vi "Close.vi"(8 "error in (no error)":errorcluster, 11 "SpinCoater in":refnum<class "SpinCoater.lvclass">) -> (0 "error out":errorcluster, 3 "SpinCoater out":refnum<class "SpinCoater.lvclass">)   [LabVIEW 2020, in "SpinCoater.lvclass"]
uses:
  <instrlib>/Classes/SpinCoater/SpinCoater.lvclass
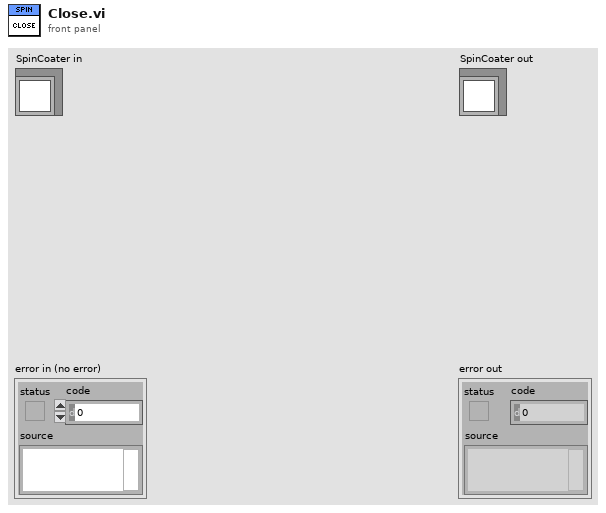
[diagram p1: front panel]
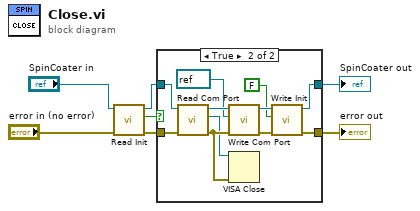
[diagram p0: block diagram]
diagram:
  n1 = call-dynamic "Read Init.vi"("error in (no error)"="error in (no error)", "SpinCoater in"="SpinCoater in") -> ("error out"=w4:errorcluster, "Init"=w3:bool, "SpinCoater out"=w5:refnum<class "SpinCoater.lvclass">)  [unwired: 7 in]
  n2 = case shown="True" w3 {
    tunnel: w5 -> [w9 w20]
    tunnel: w4 -> [w8 w19]
    tunnel: [w9 w11] -> w2
    tunnel: [w8 w10] -> w1
    frame False {
    }
    frame True {
      n3 = call-dynamic "Read Com Port.vi"("error in (no error)"=w19, "SpinCoater in"=w20) -> ("error out"=w18:errorcluster, "Com Port"=w16:refnum<visa-resource-name>, "SpinCoater out"=w17:refnum<class "SpinCoater.lvclass">)  [unwired: 7 in]
      n4 = call-dynamic "Write Com Port.vi"("error in (no error)"=w18, "Com Port"=refnum<visa-resource-name> refnum, "SpinCoater in"=w17) -> ("error out"=w13:errorcluster, "SpinCoater out"=w14:refnum<class "SpinCoater.lvclass">)  [unwired: 7 in]
      n5 = VISA Close(VISA resource name=w16, error in (no error)=w18) -> ()  [unwired: 1 out]
      n6 = call-dynamic "Write Init.vi"("error in (no error)"=w13, "Init"=FALSE, "SpinCoater in"=w14) -> ("error out"=w10:errorcluster, "SpinCoater out"=w11:refnum<class "SpinCoater.lvclass">)  [unwired: 7 in]
    }
  }
  "error out" <- w1
  "SpinCoater out" <- w2
